vi "niDTS WLAN Tx Test UTIL Static Default Parameters.vi"(10 "Standard":T2 caption="802.11 Standard") -> (2 "Static Default Parameters":T1={"Standard"=enum."802.11 n HT", "DSSS Data Rate (Mbps)"=enum."1", "OFDM Data Rate (Mbps)"=enum."54", "MCS Index"=7, "N spatial streams"=1, "Chains"=[TRUE, FALSE, FALSE, FALSE], "BandWidth (Hz)"=enum."20 MHz", "Channel"=0, "Gard Interval"=enum."SHORT", "FEC Coding"=enum."LDPC", "Dut Tx Power"=1.0, "16 symbols"=TRUE, "payload length bytes"=1500, "idle interval"=0.0001, "External Attenuation"=[0.0, 0.0, 0.0, 0.0], "Acquisition Parameters "={"Acquisition Length Mode"=enum."AUTO", "Acquisition Length (s)"=0.00015, "Auto Level"=FALSE}, "TXP Measurement Parameters"={"TXP Power Enable"=TRUE, "TXP Averages"=3}, "ModAcc Measurement Paramaters"={"ModAcc Enable"=FALSE, "Header Detection"=enum."MANUAL", "Averages"=3, "Amplitude Tracking"=FALSE, "Channel Tracking"=FALSE, "Time Tracking"=TRUE, "Phase Tracking"=enum."NONE", "Clock Offset Est"=FALSE, "Impairments Est"=FALSE, "CFO Estimation"=enum."PAMBLE"}, "ModAcc DSSS Paramaters"={"DC Offset Compensation"=TRUE, "Equalization"=TRUE, "Phase Tracking"=TRUE, "Chip Start Location"=0, "Max Chips Used"=16, "Pulse Shaping FilterType"=enum."GAUSSIAN", "Pulse Shaping Filter Coefficient"=0.35}, "SEM Measurement Parameters"={"SEM Enable"=TRUE, "SEM Averages"=3, "Auto Span Enable"=TRUE, "Frequency Span (Hz)"=66000000.0, "Measurement Type"=enum."Standard", "Mask Frequencies (Hz)"=[], "Mask Power Offsets (dB)"=[]}, "OBW Measurement Parameters"={"OBW Enable"=FALSE, "OBW Averages"=3}, "DSSS Power Ramp"={"Power Ramp Enable"=FALSE, "Averages"=3, "Thresholds"={"Up Low (%)"=10.0, "Down Low (%)"=10.0, "Up High (%)"=90.0, "Down High (%)"=90.0}}, "Enable Traces"=FALSE} {"DSSS Power Ramp"."Thresholds"."Down High (%)" min=0.0 max=100.0 step=1.0; "DSSS Power Ramp"."Thresholds"."Up High (%)" min=0.0 max=100.0 step=1.0; "DSSS Power Ramp"."Thresholds"."Down Low (%)" min=0.0 max=100.0 step=1.0; "DSSS Power Ramp"."Thresholds"."Up Low (%)" min=0.0 max=100.0 step=1.0; "Acquisition Parameters"."Acquisition Length (s)" format="%#_6p"; "SEM Measurement Parameters"."Frequency Span (Hz)" format="%#_6p"; "idle interval" format="%_3p"})   [LabVIEW 2015, in "niDTS WLAN.lvlib"]
uses:
  niDTS WLAN.lvlib
  Includes/niDTS WLAN INC Standard.ctl
  Includes/niDTS WLAN Tx Test INC Parameters.ctl
  Includes/niDTS WLAN INC DSSS Data Rate.ctl
  Includes/niDTS WLAN INC OFDM Data Rate.ctl
  Includes/niDTS WLAN INC CH BW.ctl
  Includes/niDTS WLAN INC GI.ctl
  Includes/niDTS WLAN INC FEC Coding.ctl
  Includes/niDTS WLAN DUT INC Acquisition Parameters.ctl
  Includes/niDTS WLAN INC TXP Measurement Parameters.ctl
  Includes/niDTS WLAN INC ModAcc Measurement Parameters.ctl
  Includes/niDTS WLAN INC DSSS ModAcc Measurement Parameters.ctl
  Includes/niDTS WLAN INC Pulse Shaping Filter Type.ctl
  Includes/niDTS WLAN INC SEM Measurement Parameters.ctl
  Includes/niDTS WLAN INC OBW Measurement Parameters.ctl
  Includes/niDTS WLAN INC DSSS Power Ramp Parameters.ctl
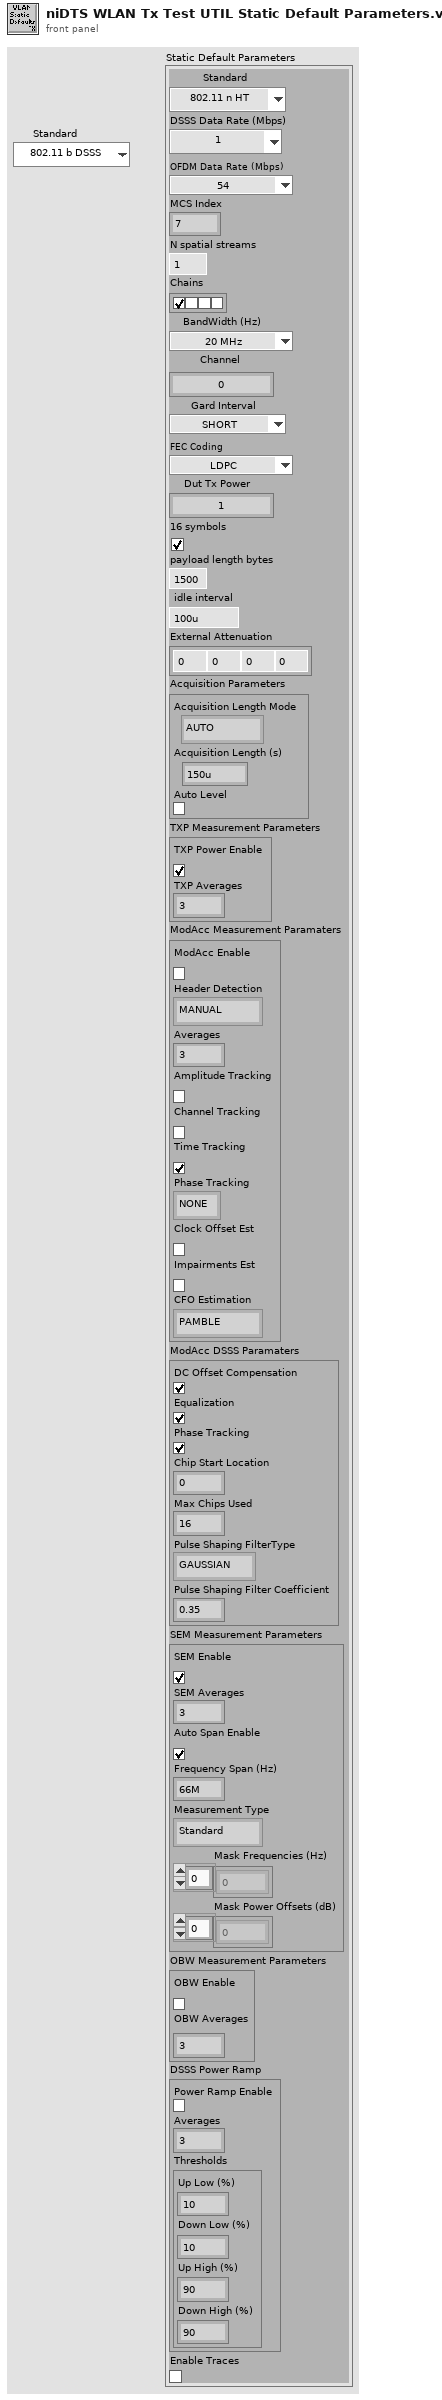
[diagram p1: front panel]
types:
  T1 = typedef "niDTS WLAN.lvlib/niDTS WLAN Tx Test INC Parameters.ctl" = cluster{"Standard":T2, "DSSS Data Rate (Mbps)":T3, "OFDM Data Rate (Mbps)":T4, "MCS Index":i32, "N spatial streams":i32, "Chains":bool[], "BandWidth (Hz)":T5, "Channel":i32, "Gard Interval":T6, "FEC Coding":T7, "Dut Tx Power":dbl, "16 symbols":bool, "payload length bytes":i32, "idle interval":dbl, "External Attenuation":dbl[], "Acquisition Parameters ":T8, "TXP Measurement Parameters":T9, "ModAcc Measurement Paramaters":T10, "ModAcc DSSS Paramaters":T11, "SEM Measurement Parameters":T13, "OBW Measurement Parameters":T14, "DSSS Power Ramp":T15, "Enable Traces":bool}
  T2 = typedef "niDTS WLAN.lvlib/niDTS WLAN INC Standard.ctl" = enum16{"802.11 b DSSS", "802.11 a/g OFDM", "802.11 n HT", "802.11 ac VHT"}
  T3 = typedef "niDTS WLAN.lvlib/niDTS WLAN INC DSSS Data Rate.ctl" = enum16{"1", "2", "5.5", "11"}
  T4 = typedef "niDTS WLAN.lvlib/niDTS WLAN INC OFDM Data Rate.ctl" = enum16{"6", "9", "12", "18", "24", "36", "48", "54"}
  T5 = typedef "niDTS WLAN.lvlib/niDTS WLAN INC CH BW.ctl" = enum16{"20 MHz", "40 MHz", "80 MHz", "160 MHz"}
  T6 = typedef "niDTS WLAN.lvlib/niDTS WLAN INC GI.ctl" = enum16{"LONG", "SHORT"}
  T7 = typedef "niDTS WLAN.lvlib/niDTS WLAN INC FEC Coding.ctl" = enum16{"BCC", "LDPC"}
  T8 = typedef "niDTS WLAN.lvlib/niDTS WLAN DUT INC Acquisition Parameters.ctl" = cluster{"Acquisition Length Mode":enum16{"AUTO", "MANUAL"}, "Acquisition Length (s)":dbl, "Auto Level":bool}
  T9 = typedef "niDTS WLAN.lvlib/niDTS WLAN INC TXP Measurement Parameters.ctl" = cluster{"TXP Power Enable":bool, "TXP Averages":i32}
  T10 = typedef "niDTS WLAN.lvlib/niDTS WLAN INC ModAcc Measurement Parameters.ctl" = cluster{"ModAcc Enable":bool, "Header Detection":enum16{"MANUAL", "FIRST", "ALL"}, "Averages":i32, "Amplitude Tracking":bool, "Channel Tracking":bool, "Time Tracking":bool, "Phase Tracking":enum16{"NONE", "STANDARD", "CSF", "INSTANT"}, "Clock Offset Est":bool, "Impairments Est":bool, "CFO Estimation":enum16{"PAMBLE", "PDATA"}}
  T11 = typedef "niDTS WLAN.lvlib/niDTS WLAN INC DSSS ModAcc Measurement Parameters.ctl" = cluster{"DC Offset Compensation":bool, "Equalization":bool, "Phase Tracking":bool, "Chip Start Location":i16, "Max Chips Used":i16, "Pulse Shaping FilterType":T12, "Pulse Shaping Filter Coefficient":dbl}
  T12 = typedef "niDTS WLAN.lvlib/niDTS WLAN INC Pulse Shaping Filter Type.ctl" = enum16{"NONE", "RCOSINE", "RRCOSINE", "GAUSSIAN"}
  T13 = typedef "niDTS WLAN.lvlib/niDTS WLAN INC SEM Measurement Parameters.ctl" = cluster{"SEM Enable":bool, "SEM Averages":i32, "Auto Span Enable":bool, "Frequency Span (Hz)":dbl, "Measurement Type":enum16{"Standard", "Legacy", "Custom"}, "Mask Frequencies (Hz)":dbl[], "Mask Power Offsets (dB)":dbl[]}
  T14 = typedef "niDTS WLAN.lvlib/niDTS WLAN INC OBW Measurement Parameters.ctl" = cluster{"OBW Enable":bool, "OBW Averages":i32}
  T15 = typedef "niDTS WLAN.lvlib/niDTS WLAN INC DSSS Power Ramp Parameters.ctl" = cluster{"Power Ramp Enable":bool, "Averages":i32, "Thresholds":cluster{"Up Low (%)":dbl, "Down Low (%)":dbl, "Up High (%)":dbl, "Down High (%)":dbl}}
  T16 = typedef "niDTS WLAN.lvlib/niDTS WLAN INC Type.ctl" = enum16{"b - 1 Mbps", "b - 2 Mbps", "b - 5.5 Mbps", "b - 11 Mbps", "ag - 6 Mbps", "ag - 9 Mbps", "ag - 12 Mbps", "ag - 18 Mbps", "ag - 24 Mbps", "ag - 36 Mbps", "ag - 48 Mbps", "ag - 54 Mbps", "n - MCS0", "n - MCS1", "n - MCS2", "n - MCS3", "n - MCS4", "n - MCS5", "n - MCS6", "n - MCS7", "n - MCS8", "n - MCS9", "n - MCS10", "n - MCS11", "n - MCS12", "n - MCS13", "n - MCS14", "n - MCS15", "n - MCS16", "n - MCS17", "n - MCS18", "n - MCS19", "n - MCS20", "n - MCS21", "n - MCS22", "n - MCS23", "n - MCS24", "n - MCS25", "n - MCS26", "n - MCS27", "n - MCS28", "n - MCS29", "n - MCS30", "n - MCS31", "ac - MCS0 -1", "ac - MCS1 -1", "ac - MCS2 -1", "ac - MCS3 -1", "ac - MCS4 -1", "ac - MCS5 -1", "ac - MCS6 -1", "ac - MCS7 -1", "ac - MCS8 -1", "ac - MCS9 -1", "ac - MCS0 -2", "ac - MCS1 -2", "ac - MCS2 -2", "ac - MCS3 -2", "ac - MCS4 -2", "ac - MCS5 -2", "ac - MCS6 -2", "ac - MCS7 -2", "ac - MCS8 -2", "ac - MCS9 -2", "ac - MCS0 -3", "ac - MCS1 -3", "ac - MCS2 -3", "ac - MCS3 -3", "ac - MCS4 -3", "ac - MCS5 -3", "ac - MCS6 -3", "ac - MCS7 -3", "ac - MCS8 -3", "ac - MCS9 -3", "ac - MCS0 -4", "ac - MCS1 -4", "ac - MCS2 -4", "ac - MCS3 -4", "ac - MCS4 -4", "ac - MCS5 -4", "ac - MCS6 -4", "ac - MCS7 -4", "ac - MCS8 -4", "ac - MCS9 -4"}
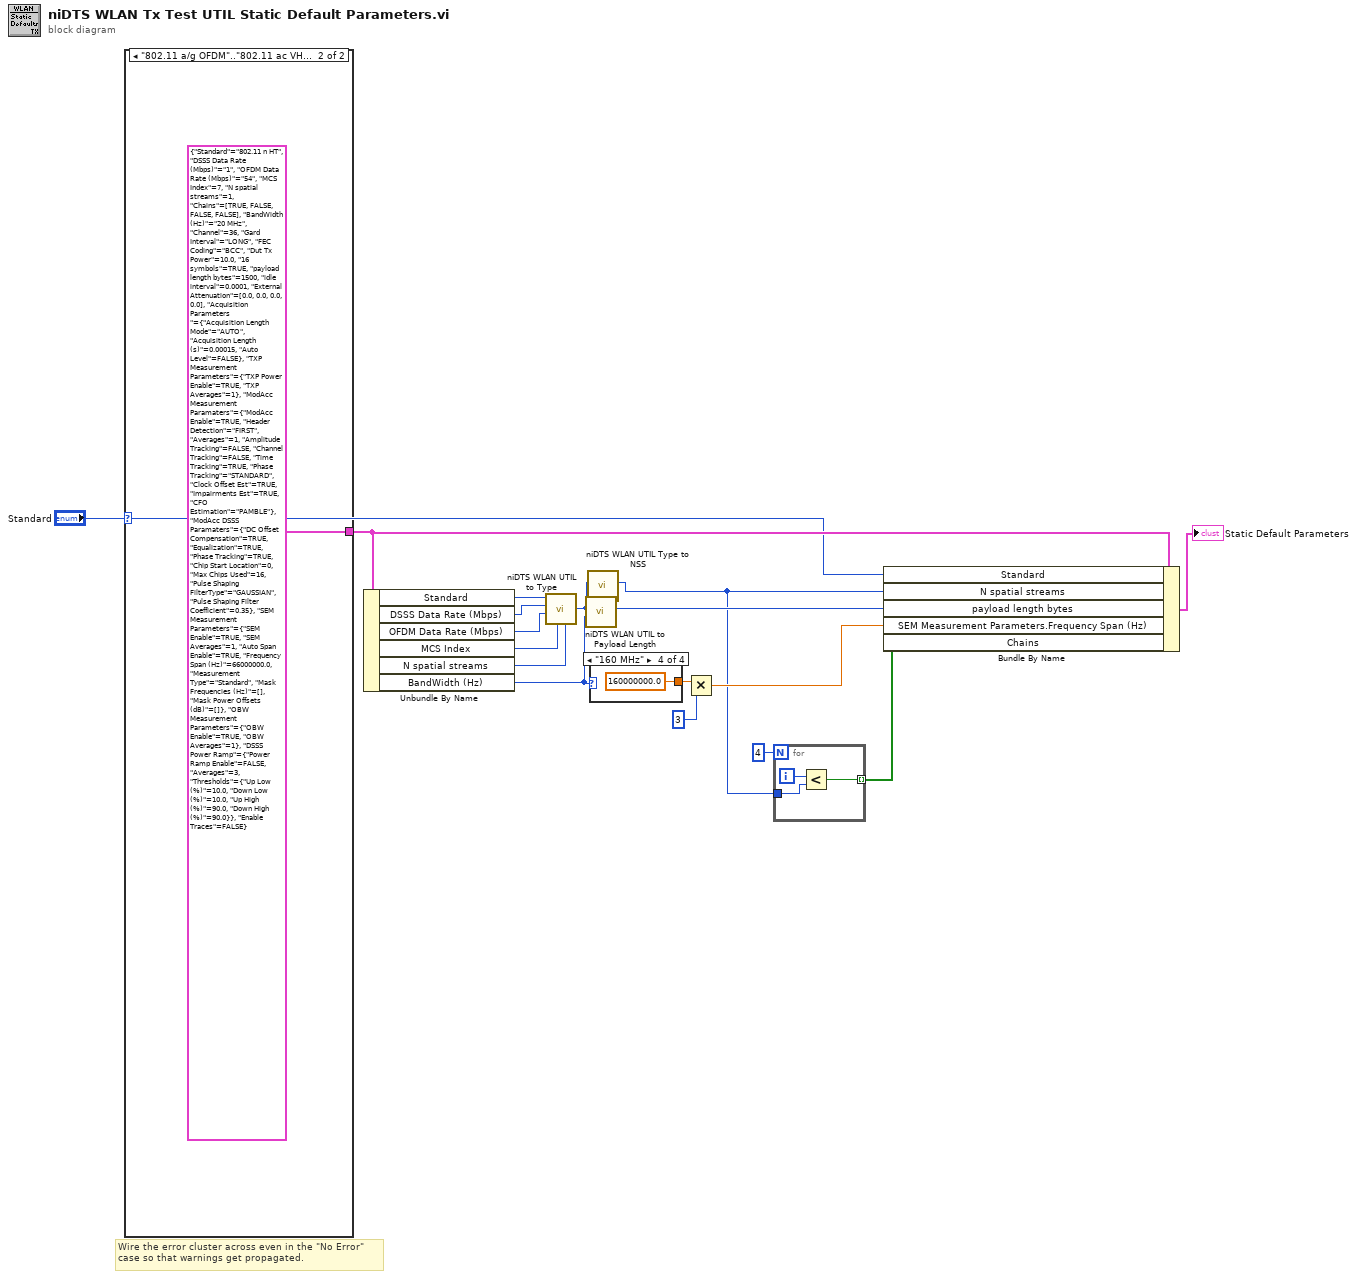
[diagram p0: block diagram]
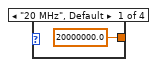
[diagram p2: hidden frame]
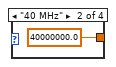
[diagram p3: hidden frame]
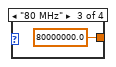
[diagram p4: hidden frame]
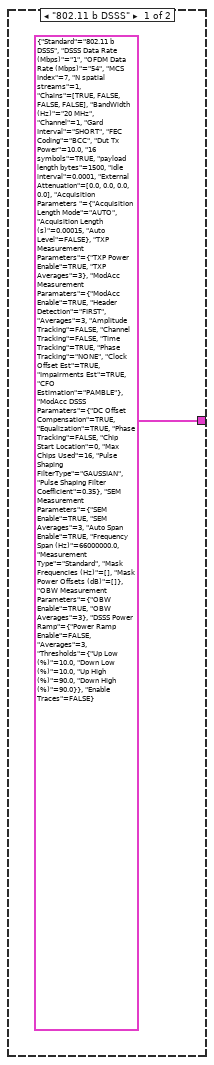
[diagram p5: hidden frame]
diagram:
  # "Wire the error cluster across even in the \"No Error\"\ncase so that warnings get propagated."
  n1 = case shown="\"802.11 a/g OFDM\"..\"802.11 ac VHT\", Default" "Standard" {
    tunnel: [T1 {"Standard"=enum."802.11 b DSSS", "DSSS Data Rate (Mbps)"=enum."1", "OFDM Data Rate (Mbps)"=enum."54", "MCS Index"=7, "N spatial streams"=1, "Chains"=[TRUE, FALSE, FALSE, FALSE], "BandWidth (Hz)"=enum."20 MHz", "Channel"=1, "Gard Interval"=enum."SHORT", "FEC Coding"=enum."BCC", "Dut Tx Power"=10.0, "16 symbols"=TRUE, "payload length bytes"=1500, "idle interval"=0.0001, "External Attenuation"=[0.0, 0.0, 0.0, 0.0], "Acquisition Parameters "={"Acquisition Length Mode"=enum."AUTO", "Acquisition Length (s)"=0.00015, "Auto Level"=FALSE}, "TXP Measurement Parameters"={"TXP Power Enable"=TRUE, "TXP Averages"=3}, "ModAcc Measurement Paramaters"={"ModAcc Enable"=TRUE, "Header Detection"=enum."FIRST", "Averages"=3, "Amplitude Tracking"=FALSE, "Channel Tracking"=FALSE, "Time Tracking"=TRUE, "Phase Tracking"=enum."NONE", "Clock Offset Est"=TRUE, "Impairments Est"=TRUE, "CFO Estimation"=enum."PAMBLE"}, "ModAcc DSSS Paramaters"={"DC Offset Compensation"=TRUE, "Equalization"=TRUE, "Phase Tracking"=FALSE, "Chip Start Location"=0, "Max Chips Used"=16, "Pulse Shaping FilterType"=enum."GAUSSIAN", "Pulse Shaping Filter Coefficient"=0.35}, "SEM Measurement Parameters"={"SEM Enable"=TRUE, "SEM Averages"=3, "Auto Span Enable"=TRUE, "Frequency Span (Hz)"=66000000.0, "Measurement Type"=enum."Standard", "Mask Frequencies (Hz)"=[], "Mask Power Offsets (dB)"=[]}, "OBW Measurement Parameters"={"OBW Enable"=TRUE, "OBW Averages"=3}, "DSSS Power Ramp"={"Power Ramp Enable"=FALSE, "Averages"=3, "Thresholds"={"Up Low (%)"=10.0, "Down Low (%)"=10.0, "Up High (%)"=90.0, "Down High (%)"=90.0}}, "Enable Traces"=FALSE} ("Static Default Parameters") T1 {"Standard"=enum."802.11 n HT", "DSSS Data Rate (Mbps)"=enum."1", "OFDM Data Rate (Mbps)"=enum."54", "MCS Index"=7, "N spatial streams"=1, "Chains"=[TRUE, FALSE, FALSE, FALSE], "BandWidth (Hz)"=enum."20 MHz", "Channel"=36, "Gard Interval"=enum."LONG", "FEC Coding"=enum."BCC", "Dut Tx Power"=10.0, "16 symbols"=TRUE, "payload length bytes"=1500, "idle interval"=0.0001, "External Attenuation"=[0.0, 0.0, 0.0, 0.0], "Acquisition Parameters "={"Acquisition Length Mode"=enum."AUTO", "Acquisition Length (s)"=0.00015, "Auto Level"=FALSE}, "TXP Measurement Parameters"={"TXP Power Enable"=TRUE, "TXP Averages"=1}, "ModAcc Measurement Paramaters"={"ModAcc Enable"=TRUE, "Header Detection"=enum."FIRST", "Averages"=1, "Amplitude Tracking"=FALSE, "Channel Tracking"=FALSE, "Time Tracking"=TRUE, "Phase Tracking"=enum."STANDARD", "Clock Offset Est"=TRUE, "Impairments Est"=TRUE, "CFO Estimation"=enum."PAMBLE"}, "ModAcc DSSS Paramaters"={"DC Offset Compensation"=TRUE, "Equalization"=TRUE, "Phase Tracking"=TRUE, "Chip Start Location"=0, "Max Chips Used"=16, "Pulse Shaping FilterType"=enum."GAUSSIAN", "Pulse Shaping Filter Coefficient"=0.35}, "SEM Measurement Parameters"={"SEM Enable"=TRUE, "SEM Averages"=1, "Auto Span Enable"=TRUE, "Frequency Span (Hz)"=66000000.0, "Measurement Type"=enum."Standard", "Mask Frequencies (Hz)"=[], "Mask Power Offsets (dB)"=[]}, "OBW Measurement Parameters"={"OBW Enable"=TRUE, "OBW Averages"=1}, "DSSS Power Ramp"={"Power Ramp Enable"=FALSE, "Averages"=3, "Thresholds"={"Up Low (%)"=10.0, "Down Low (%)"=10.0, "Up High (%)"=90.0, "Down High (%)"=90.0}}, "Enable Traces"=FALSE} ("Static Default Parameters")] -> w17
    frame "802.11 b DSSS" {
    }
    frame "802.11 a/g OFDM".."802.11 ac VHT", Default {
    }
  }
  n2 = Unbundle By Name(w17) -> ("Standard"=w7:T2, "DSSS Data Rate (Mbps)"=w14:T3, "OFDM Data Rate (Mbps)"=w13:T4, "MCS Index"=w6:i32, "N spatial streams"=w5:i32, "BandWidth (Hz)"=w11:T5)
  n3 = call "niDTS WLAN UTIL to Type.vi"("N_SS"=w5, "MCS"=w6, "OFDM Data Rate (Mbps)"=w13, "DSSS Data Rate (Mbps)"=w14, "Standard"=w7) -> ("WLAN Type"=w4:T16)  [unwired: 6 in]
  n4 = call "niDTS WLAN UTIL to Payload Length.vi"("CH BW"=w11, "WLAN Type"=w4) -> ("Payload Length"=w16:i32)  [unwired: 9 in]
  n5 = call "niDTS WLAN UTIL Type to NSS.vi"("WLAN Type"=w4) -> ("NSS"=w2:i32)  [unwired: 10 in]
  n6 = case shown="\"160 MHz\"" w11 {
    tunnel: [20000000.0 ("FrequencySpan") 40000000.0 ("FrequencySpan") 80000000.0 ("FrequencySpan") 160000000.0 ("FrequencySpan")] -> w10
    frame "20 MHz", Default {
    }
    frame "40 MHz" {
    }
    frame "80 MHz" {
    }
    frame "160 MHz" {
    }
  }
  n7 = Multiply(x=w10, y=3) -> (x*y=w8:dbl)
  n8 = for {
    N: 4 -> [_]
    tunnel: w2 -> [w25]
    tunnel: [w24] -> w1 mode=indexing
    i -> [w26]
    n9 = Less?(x=w26, y=w25) -> (x < y?=w24:bool)
  }
  n10 = Bundle By Name(cluster=w17, "Standard"="Standard", "N spatial streams"=w2, "payload length bytes"=w16, "SEM Measurement Parameters.Frequency Span (Hz)"=w8, "Chains"=w1) -> (→"Static Default Parameters":T1)
